vi "nanocal--mathstring--load   -- V1.vi"(0 "mathstring IN":string, 2 "MAIN folder":path=path "Users/arkadyshekhter/Library/CloudStorage/Dropbox/shared_AkashAndreas/paper-CeCoIn5-spectroheat/Original RAW data", 5 "side map to STR":map{T1, string}(c390), 7 "side map to NUM":map{T1, i32}(c390), 9 "data file parameters map":map{T2, T3}(c390), 11 "what? IN":T4 {"B (T)" items=["0.000", "1.000", "2.000", "4.000", "5.000", "6.000", "7.000", "8.000", "9.000", "10.000", "11.000", "12.000"]; "θ (∘)" items=["0.000", "30.000", "45.000", "60.000", "90.000"]; "T (K)" items=["0.120", "0.122", "0.140", "0.148", "0.150", "0.157", "0.160", "0.168", "0.170", "0.178", "0.179", "0.180", "0.190", "0.197", "0.200", "0.249", "0.250", "0.255", "0.260", "0.300", "0.307", "0.308", "0.310", "0.360", "0.420", "0.430", "0.438", "0.512", "0.520", "0.530", "0.610", "0.620", "0.630", "0.677", "0.810", "0.820", "0.830", "1.000", "1.100", "1.120", "1.130", "1.250", "1.280", "1.310", "1.390", "1.500", "1.520", "1.550", "1.600", "1.700", "1.800", "1.900", "2.100", "2.300", "3.000", "3.070", "3.100", "3.110", "5.500", "5.700", "5.750"]; "side (8S|4R)" items=["4000", "8000"]; "set (1T|2B)" items=["1", "2"]}, 13 "data file pattern":string="IDS*RAW*_raw_.dat") -> (4 "all short filenames":map{string, string}(c390), 6 "temps&degs":map{string, map{T2, dbl}}(c390), 8 "mathematica thing":map{string, map{T2, dbl}}(c390), 10 "all full filenames":map{string, path}(c390), 15 "what? OUT":T4 {"B (T)" items=["0.000", "1.000", "2.000", "4.000", "5.000", "6.000", "7.000", "8.000", "9.000", "10.000", "11.000", "12.000"]; "θ (∘)" items=["0.000", "30.000", "45.000", "60.000", "90.000"]; "T (K)" items=["0.120", "0.122", "0.140", "0.148", "0.150", "0.157", "0.160", "0.168", "0.170", "0.178", "0.179", "0.180", "0.190", "0.197", "0.200", "0.249", "0.250", "0.255", "0.260", "0.300", "0.307", "0.308", "0.310", "0.360", "0.420", "0.430", "0.438", "0.512", "0.520", "0.530", "0.610", "0.620", "0.630", "0.677", "0.810", "0.820", "0.830", "1.000", "1.100", "1.120", "1.130", "1.250", "1.280", "1.310", "1.390", "1.500", "1.520", "1.550", "1.600", "1.700", "1.800", "1.900", "2.100", "2.300", "3.000", "3.070", "3.100", "3.110", "5.500", "5.700", "5.750"]; "side (8S|4R)" items=["4000", "8000"]; "set (1T|2B)" items=["1", "2"]})   [LabVIEW 2021]
uses:
  3-lorentzian-parameters.ctl
  nanocal_side_selector.ctl
  filename-action.ctl
  3-lorentzian-heat-response action.ctl
  <vilib>/Utility/miscctls.llb/LVMapReplaceAction.ctl
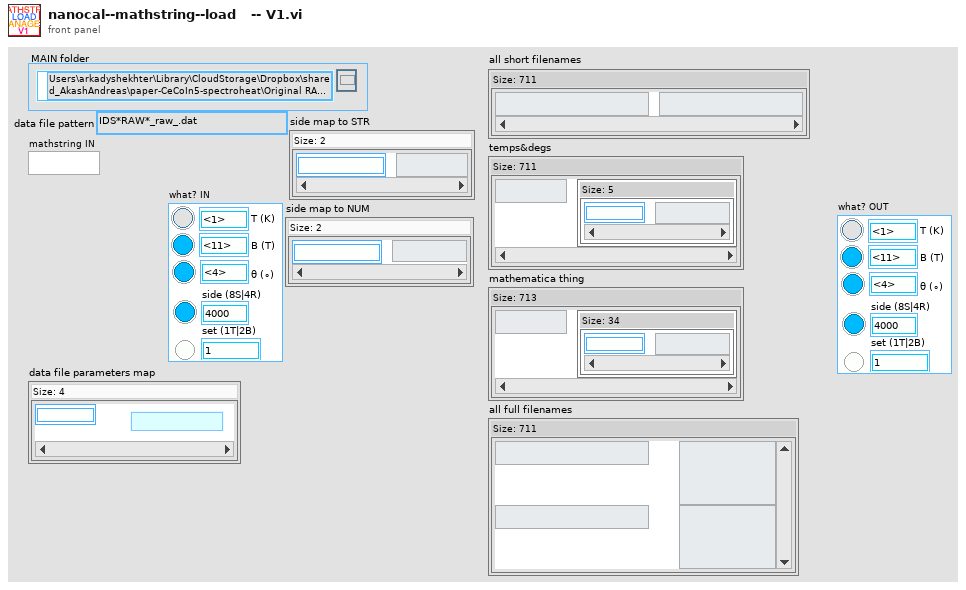
[diagram p1: front panel]
types:
  T1 = typedef "nanocal_side_selector.ctl" = enum16{"sam", "ref"}
  T2 = typedef "3-lorentzian-parameters.ctl" = enum16{"ζ", "τ1", "τS", "τN", "τC", "κ0", "m1", "m2", "m3", "T (K)", "B (T)", "θ (deg)", "side (S|R)", "set of (B|T)", "Re(offset)", "Im(offset)", "στ1", "στ1-", "στ1+", "στS", "στS-", "στS+", "στN", "στN-", "στN+", "τ11", "τ12", "τ21", "τ22", "τN1", "τN2", "σηlogτ1", "σηlogτS", "σηlogτN", "σlogτ1", "σlogτS", "σlogτN", "σητ1", "σητS", "σητN", "noiseT"}
  T3 = typedef "filename-action.ctl" = enum16{"rewrite", "parse", "force pattern", "uniquenum", "get T", "get B", "get ind", "get deg", "get name", "get folder", "get extension", "get basename", "get side", "get setof", "getID", "getIDStock"}
  T4 = cluster{"ignore set of !":bool, "set (1T|2B)":i32, "ignore side !":bool, "side (8S|4R)":i64, "ignore θ !":bool, "ignore B !":bool, "T (K)":dbl, "ignore T !":bool, "θ (∘)":dbl, "B (T)":dbl, "lookup":cluster{"set of lookup":map{i32, dbl}, "all set of":set{dbl}, "T lookup":map{i32, dbl}, "θ lookup":map{i32, dbl}, "B lookup":map{i32, dbl}, "all T's":set{dbl}, "all θ's":set{dbl}, "all B's":set{dbl}, "all sides":set{dbl}, "side lookup":map{i32, dbl}}}
  T5 = typedef "3-lorentzian-heat-response action.ctl" = enum16{"calc R", "create string", "calc m1m2m3", "dζ", "dT1", "dτS", "dτN", "dτC", "d-all", "dκ0", "T(K)", "m1", "m2", "m3", "parse string", "θ (deg)", "B (T)", "onlygrads", "newton", "create emty string", "simple2nd", "calc R2", "ScalarProd", "ScalarProd-diff", "nothing", "ScalarProd-eta", "tolog", "ignore", "three2nd", "eta-errors"}
  T6 = typedef "LVMapReplaceAction.ctl" = enum32{"Modify Entry only if found", "Add or Modify Entry", "Delete Entry"}
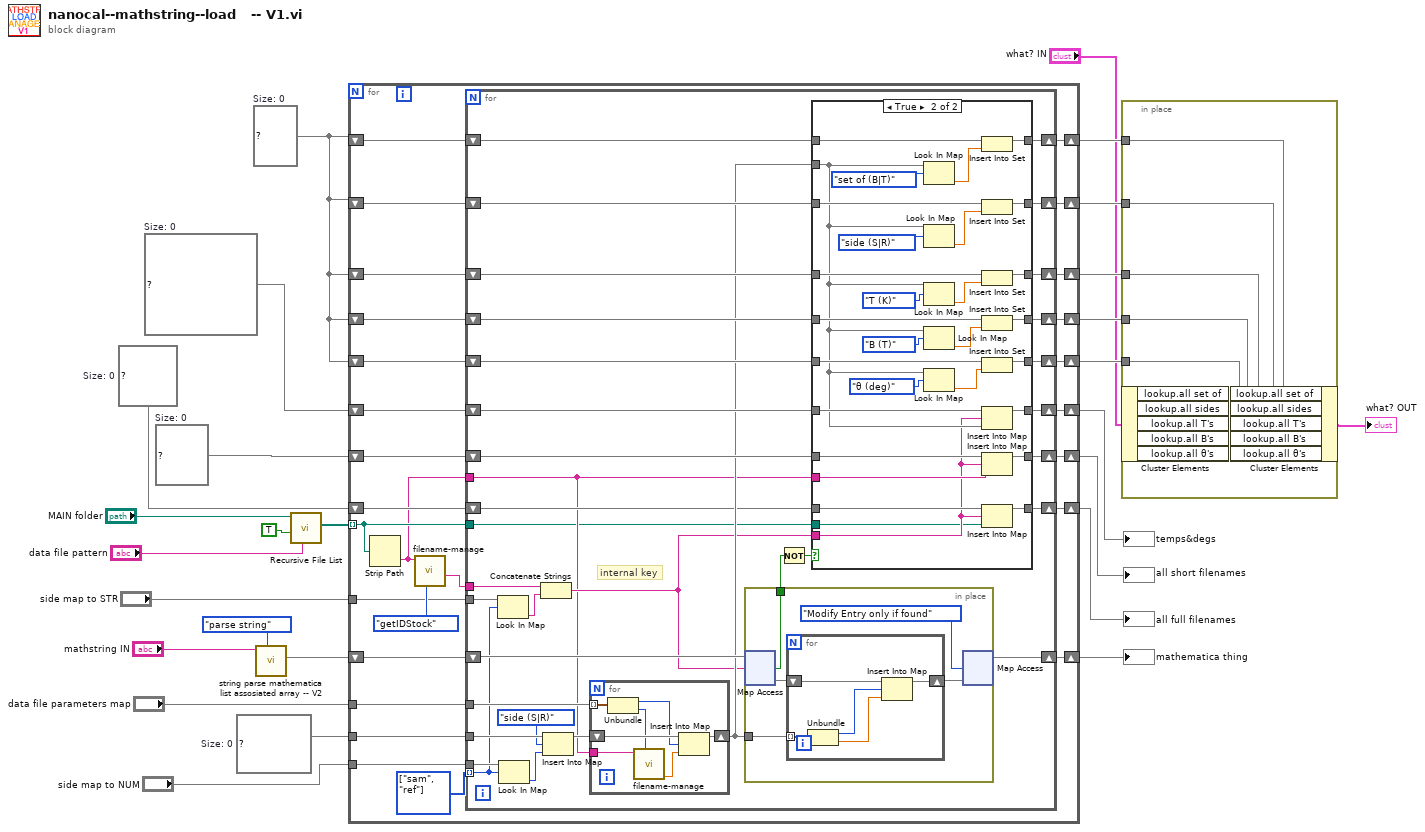
[diagram p0: block diagram]
diagram:
  w16 = map{string, path} {}  # Size: 0
  w24 = map{T2, dbl} {}  # Size: 0
  w23 = set{dbl} {}  # Size: 0
  w25 = map{string, map{T2, dbl}} {}  # Size: 0
  w20 = map{string, string} {}  # Size: 0
  n1 = call "string parse mathematica list assosiated array -- V2.vi"("action"=3-lorentzian-heat-response_action."parse string" ("derivative"), "string IN"="mathstring IN") -> ("all keys Map OUT"=w26:map{string, map{T2, dbl}})  [unwired: 6 in, 3 out]
  n2 = call <vilib>:"Recursive File List.vi"("pattern"="data file pattern", "Continue Recursing on Error? (F)"=TRUE, "Folder Path"="MAIN folder") -> ("All Files in Dir"=w17:path[])  [unwired: 4 in, 4 out]
  n3 = for {
    tunnel: w17 -> [w28] mode=indexing
    shift-right: [w42] -> w9
    shift-left: w26 -> [w52]
    shift-right: [w39] -> w22
    shift-left: w20 -> [w51]
    shift-right: [w38] -> w21
    shift-left: w25 -> [w47]
    shift-right: [w49] -> w13
    shift-left: w23 -> [w41]
    shift-right: [w40] -> w12
    shift-left: w23 -> [w50]
    tunnel: w24 -> [w45]
    shift-right: [w35] -> w11
    shift-left: w23 -> [w48]
    shift-right: [w37] -> w14
    shift-left: w23 -> [w46]
    tunnel: "data file parameters map" -> [w44]
    shift-right: [w36] -> w15
    shift-left: w23 -> [w43]
    tunnel: "side map to NUM" -> [w33]
    tunnel: "side map to STR" -> [w32]
    shift-right: [w29] -> w19
    shift-left: w16 -> [w30]
    w31 = T1[] [enum."sam", enum."ref"] items=["sam", "ref"]
    n4 = Strip Path(path=w28) -> (name=w27:string)  [unwired: 1 out]
    n5 = call "filename-manage.vi"("filename-action"=filename-action."getIDStock", "file name IN"=w27) -> ("string OUT"=w34:string)  [unwired: 7 in, 2 out]
    n6 = for {
      tunnel: w44 -> [w78]
      tunnel: w27 -> [w55]
      tunnel: w34 -> [w67]
      shift-right: [w76] -> w42
      shift-left: w52 -> [w87]
      shift-right: [w82] -> w49
      shift-left: w41 -> [w75]
      shift-right: [w74] -> w40
      shift-left: w50 -> [w83]
      shift-right: [w68] -> w35
      shift-left: w48 -> [w81]
      shift-right: [w69] -> w37
      shift-left: w46 -> [w79]
      shift-right: [w70] -> w36
      shift-left: w43 -> [w77]
      shift-right: [w71] -> w38
      shift-left: w47 -> [w80]
      shift-right: [w72] -> w39
      shift-left: w51 -> [w86]
      tunnel: w33 -> [w60]
      tunnel: w45 -> [w65]
      tunnel: w32 -> [w62]
      tunnel: w31 -> [w59] mode=indexing
      shift-right: [w56] -> w29
      shift-left: w30 -> [w57]
      tunnel: w28 -> [w54]
      # "internal key"
      n7 = Look In Map(map=w62, key=w59) -> (value=w61:string)  [unwired: 1 in, 1 out]
      n8 = Look In Map(map=w60, key=w59) -> (value=w58:i32)  [unwired: 1 in, 1 out]
      n9 = Concatenate Strings(w67, w61) -> (w66:string)
      n10 = Insert Into Map(map in=w65, key=3-lorentzian-parameters."side (S|R)", value=w58) -> (map out=w64:map{T2, dbl})  [unwired: 2 out]
      n11 = for {
        shift-right: [w93] -> w73
        shift-left: w64 -> [w94]
        tunnel: w78 -> [w92] mode=indexing
        tunnel: w55 -> [w90]
        n12 = Unbundle(w92) -> ("key"=w91:T2, "filename-action"=w89:T3)
        n13 = call "filename-manage.vi"("filename-action"=w89, "file name IN"=w90) -> ("number OUT"=w88:dbl)  [unwired: 7 in, 2 out]
        n14 = Insert Into Map(map in=w94, key=w91, value=w88) -> (map out=w93:map{T2, dbl})  [unwired: 2 out]
      }
      n15 = in-place {
        in-place-border: [w136] -> w85
        in-place-border: w73 -> [w135]
        n16 = in-place-map #1(w87, w66) -> (w134:map{T2, dbl}, w136:bool)  [unwired: 1 in]
        n17 = for {
          tunnel: w135 -> [w142] mode=indexing
          shift-right: [w140] -> w133
          shift-left: w134 -> [w141]
          n18 = Unbundle(w142) -> ("key"=w139:T2, "number OUT"=w138:dbl)
          n19 = Insert Into Map(map in=w141, key=w139, value=w138) -> (map out=w140:map{T2, dbl})  [unwired: 2 out]
        }
        n20 = in-place-map #1(w133, LVMapReplaceAction."Modify Entry only if found" ("action")) -> (w76:map{string, map{T2, dbl}})  [unwired: 2 out]
      }
      n21 = Not(x=w85) -> (.not. x?=w84:bool)
      n22 = case shown="True" w84 {
        tunnel: w86 -> [w102 w132]
        tunnel: [w102 w131] -> w72
        tunnel: w55 -> [_ w130]
        tunnel: w66 -> [_ w104]
        tunnel: w83 -> [w100 w129]
        tunnel: [w100 w128] -> w74
        tunnel: w75 -> [w101 w127]
        tunnel: [w101 w126] -> w82
        tunnel: [w98 w125] -> w68
        tunnel: w81 -> [w98 w124]
        tunnel: w73 -> [_ w109]
        tunnel: w80 -> [w99 w123]
        tunnel: [w99 w122] -> w71
        tunnel: [w97 w121] -> w69
        tunnel: w79 -> [w97 w120]
        tunnel: [w96 w111] -> w70
        tunnel: w77 -> [w96 w110]
        tunnel: w57 -> [w95 w106]
        tunnel: [w95 w105] -> w56
        tunnel: w54 -> [_ w103]
        frame False {
        }
        frame True {
          n23 = Look In Map(map=w109, key=3-lorentzian-parameters."set of (B|T)") -> (value=w112:dbl)  [unwired: 1 in, 1 out]
          n24 = Look In Map(map=w109, key=3-lorentzian-parameters."side (S|R)") -> (value=w118:dbl)  [unwired: 1 in, 1 out]
          n25 = Look In Map(map=w109, key=3-lorentzian-parameters."T (K)") -> (value=w116:dbl)  [unwired: 1 in, 1 out]
          n26 = Look In Map(map=w109, key=3-lorentzian-parameters."B (T)") -> (value=w108:dbl)  [unwired: 1 in, 1 out]
          n27 = Look In Map(map=w109, key=3-lorentzian-parameters."θ (deg)") -> (value=w107:dbl)  [unwired: 1 in, 1 out]
          n28 = Insert Into Set(10:w112, 11:w110) -> (3:w111:set{dbl})  [unwired: 1 out]
          n29 = Insert Into Set(10:w118, 11:w120) -> (3:w121:set{dbl})  [unwired: 1 out]
          n30 = Insert Into Set(10:w116, 11:w124) -> (3:w125:set{dbl})  [unwired: 1 out]
          n31 = Insert Into Set(10:w108, 11:w129) -> (3:w128:set{dbl})  [unwired: 1 out]
          n32 = Insert Into Set(10:w107, 11:w127) -> (3:w126:set{dbl})  [unwired: 1 out]
          n33 = Insert Into Map(map in=w123, key=w104, value=w109) -> (map out=w122:map{string, map{T2, dbl}})  [unwired: 2 out]
          n34 = Insert Into Map(map in=w132, key=w104, value=w130) -> (map out=w131:map{string, string})  [unwired: 2 out]
          n35 = Insert Into Map(map in=w106, key=w104, value=w103) -> (map out=w105:map{string, path})  [unwired: 2 out]
        }
      }
    }
  }
  "all short filenames" <- w22
  "temps&degs" <- w21
  "mathematica thing" <- w9
  "all full filenames" <- w19
  n36 = in-place {
    in-place-border: w15 -> [w147]
    in-place-border: w14 -> [w146]
    in-place-border: w13 -> [w143]
    in-place-border: w12 -> [w144]
    in-place-border: w11 -> [w145]
    n37 = in-place-cluster #2("what? IN") -> ()  [unwired: 5 out]
    n38 = in-place-cluster #2("lookup.all set of"=w147, "lookup.all sides"=w146, "lookup.all T's"=w145, "lookup.all B's"=w144, "lookup.all θ's"=w143) -> (→"what? OUT":T4)
  }
